vi "Ball Update.vi"(5 "Direction in":cluster{"x_dir":i32, "y_dir":i32}, 6 "Ball Ref":refnum<vi>, 7 "AreaSize":T1) -> (0 "LostBall":bool, 1 "Direction":cluster{"x_dir":i32, "y_dir":i32}, 2 "Ball Center":T2, 3 "Ball ref out":refnum<vi>)   [LabVIEW 8.6]
uses:
  VI_Control/Ball Center Ctrl.ctl
  <vilib>/Utility/miscctls.llb/LVBoundsTypeDef.ctl
panel:
  in  "Ball":bool
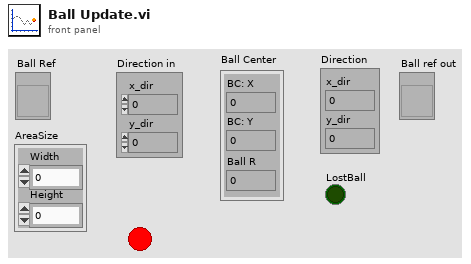
[diagram p1: front panel]
types:
  T1 = typedef "LVBoundsTypeDef.ctl" = cluster{"Width":u32, "Height":u32}
  T2 = typedef "Ball Center Ctrl.ctl" = cluster{"BC: X":i32, "BC: Y":i32, "Ball R":i32}
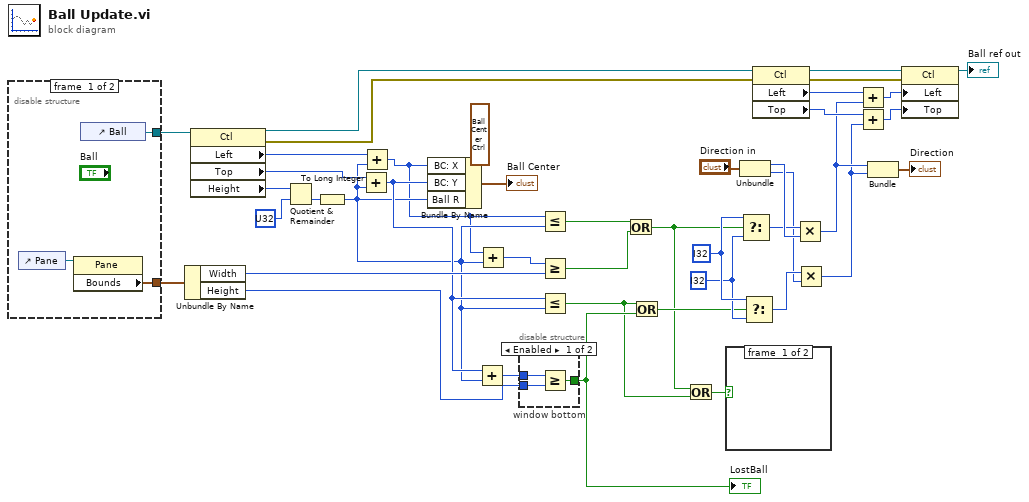
[diagram p0: block diagram]
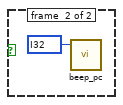
[diagram p2: hidden frame]
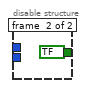
[diagram p3: hidden frame]
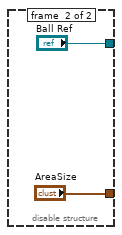
[diagram p4: hidden frame]
diagram:
  w26 = i32 ?
  w27 = i32 ?
  n1 = disable-structure shown="Enabled" {
    disable-tunnel: [w45 "Ball Ref"] -> w29
    disable-tunnel: [w43 "AreaSize"] -> w10
    frame #0 {
      n2 = control-ref of="Pane"() -> (w44:refnum<vi>)
      n3 = property class="Pane"(reference=w44) -> ("Bounds"=w43:T1)  [unwired: 1 in, 2 out]
      n4 = control-ref of="Ball"() -> (w45:refnum<vi>)
    }
    frame #1 {
    }
  }
  n5 = Unbundle By Name(w10) -> ("Width"=w9:u32, "Height"=w8:u32)
  n6 = property class="Ctl"(reference=w29) -> (reference out=w18:refnum<vi>, error out=w12:errorcluster, "Left"=w41:i32, "Top"=w40:i32, "Height"=w38:u32)  [unwired: 1 in]
  n7 = Quotient & Remainder(x=w38, y=u32 ?) -> (floor(x/y)=w37:u32)  [unwired: 1 out]
  n8 = To Long Integer(number=w37) -> (32bit integer=w5:i32)
  n9 = Add(x=w40, y=w5) -> (x+y=w6:i32)
  n10 = Add(x=w41, y=w5) -> (x+y=w4:i32)
  n11 = Bundle By Name(cluster=T2 ? ("Ball Center"), "BC: X"=w4, "BC: Y"=w6, "Ball R"=w5) -> (→"Ball Center":T2)
  n12 = Add(x=w6, y=w5) -> (x+y=w31:i32)
  n13 = Add(x=w4, y=w5) -> (x+y=w35:i32)
  n14 = disable-structure "window bottom" shown="Enabled" {
    disable-tunnel: [w50 bool ?] -> w32
    disable-tunnel: w31 -> [w49 _]
    disable-tunnel: w8 -> [w48 _]
    frame #0 {
      n15 = Greater Or Equal?(x=w49, y=w48) -> (x >= y?=w50:bool)
    }
    frame #1 {
    }
  }
  "LostBall" <- w32
  n16 = Less Or Equal?(x=w4, y=w5) -> (x <= y?=w36:bool)
  n17 = Greater Or Equal?(x=w35, y=w9) -> (x >= y?=w34:bool)
  n18 = Less Or Equal?(x=w6, y=w5) -> (x <= y?=w2:bool)
  n19 = Or(x=w36, y=w34) -> (x .or. y?=w3:bool)
  n20 = Or(x=w2, y=w32) -> (x .or. y?=w25:bool)
  n21 = Or(x=w3, y=w2) -> (x .or. y?=w1:bool)
  n22 = case shown="True" w1 {
    frame #0 {
    }
    frame #1 {
      n23 = call "beep_pc.vi"("Frequency (Hz)"=i32 ?) -> ()  [unwired: 3 in, 1 out]
    }
  }
  n24 = Unbundle("Direction in") -> ("x_dir"=w24:i32, "y_dir"=w21:i32)
  n25 = Select(t=w27, s=w3, f=w26) -> (s? t:f=w23:i32)
  n26 = Select(t=w27, s=w25, f=w26) -> (s? t:f=w22:i32)
  n27 = property class="Ctl"(reference=w18, error in=w12) -> (reference out=w13:refnum<vi>, error out=w11:errorcluster, "Left"=w17:i32, "Top"=w16:i32)
  n28 = Multiply(x=w23, y=w24) -> (x*y=w15:i32)
  n29 = Multiply(x=w22, y=w21) -> (x*y=w14:i32)
  n30 = Add(x=w17, y=w15) -> (x+y=w20:i32)
  n31 = Add(x=w16, y=w14) -> (x+y=w19:i32)
  n32 = Bundle(w15, w14) -> (→"Direction":cluster{i32, i32})  [unwired: 1 in]
  n33 = property class="Ctl"(reference=w13, error in=w11, "Left"=w20, "Top"=w19) -> (reference out=→"Ball ref out":refnum<vi>)  [unwired: 1 out]
